vi "Select DB.vi"() -> (0 "Cancel out":bool, 1 "Invert Channels out":bool, 2 "XNET Database out":refnum<k21>)   [LabVIEW 2017, in "J1939 editor node.lvclass"]
uses:
  J1939 editor node.lvclass
panel:
  in  "Cancel":bool
  in  "OK":bool
  in  "Invert Channels?":bool
  in  "XNET Database":refnum<k21>
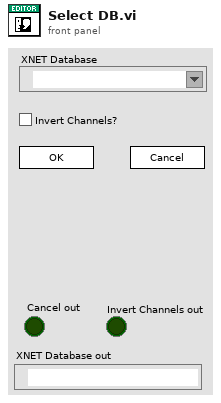
[diagram p1: front panel]
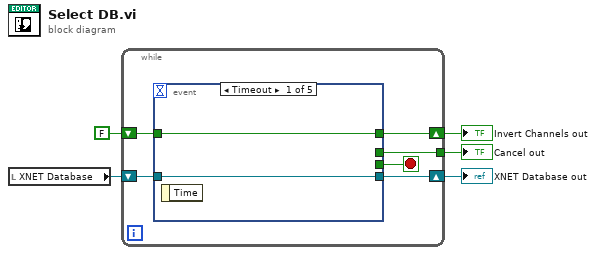
[diagram p0: block diagram]
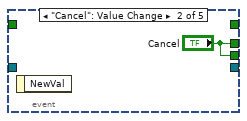
[diagram p2: hidden frame]
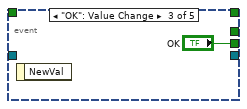
[diagram p3: hidden frame]
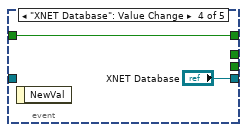
[diagram p4: hidden frame]
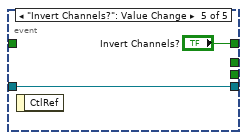
[diagram p5: hidden frame]
diagram:
  n1 = local read "XNET Database"() -> (w5:refnum<k21>)
  n2 = while {
    shift-right: [w11] -> w1
    shift-left: w5 -> [w10]
    shift-right: [w9] -> w2
    shift-left: FALSE ("Invert Channels?") -> [w8]
    tunnel: [w7] -> w3
    stop <- w6 stop-if-true
    n3 = event shown="[0] Timeout" {
      selector: _ -> [_ _ _ _ _]
      dyn-events: _ -> [_ _ _ _ _]
      timeout: _ -> [_ _ _ _ _]
      tunnel: [w13 _ _ "XNET Database" w19] -> w11
      tunnel: w10 -> [w13 _ _ _ w19]
      tunnel: [w12 _ _ w16 "Invert Channels?"] -> w9
      tunnel: w8 -> [w12 _ _ w16 _]
      tunnel: [_ "Cancel" _ _ _] -> w7
      tunnel: [_ "Cancel" "OK" _ _] -> w6
      event Timeout {
        n4 = event-data() -> ()  [unwired: 1 in, 1 out]
      }
      event "Cancel": Value Change {
        n5 = event-data() -> ()  [unwired: 1 in, 1 out]
      }
      event "OK": Value Change {
        n6 = event-data() -> ()  [unwired: 1 in, 1 out]
      }
      event "XNET Database": Value Change {
        n7 = event-data() -> ()  [unwired: 1 in, 1 out]
      }
      event "Invert Channels?": Value Change {
        n8 = event-data() -> ()  [unwired: 1 in, 1 out]
      }
    }
  }
  "Cancel out" <- w3
  "Invert Channels out" <- w2
  "XNET Database out" <- w1
